vi "Fire DAQStateChanged Event_DAQ.vi"(8 "error in (no error)":errorcluster, 9 "vData":variant, 10 "DAQState":variant, 11 "DAQ":refnum<class "DAQ.lvclass">) -> (0 "error out":errorcluster, 3 "DAQ out":refnum<class "DAQ.lvclass">)   [LabVIEW 2017, in "DAQ.lvclass"]
doc: "Developed by Kevin Thompson\nkevin@thompsonengineering.net\n\nCopyright 2018-2020\nThompson Engineering, LLC"
uses:
  DAQ.lvclass
  DataTypes/TD DAQStateChanged EventData--cluster.ctl
  DataTypes/TD DAQ&TDMS State Data--cluster.ctl
  DataTypes/TD DaqState--enum.ctl
  DAQ.lvclass/DAQ.ctl
  Accessors/Get DAQ&TDMS State Data.vi
  Accessors/Set DAQ&TDMS State Data.vi
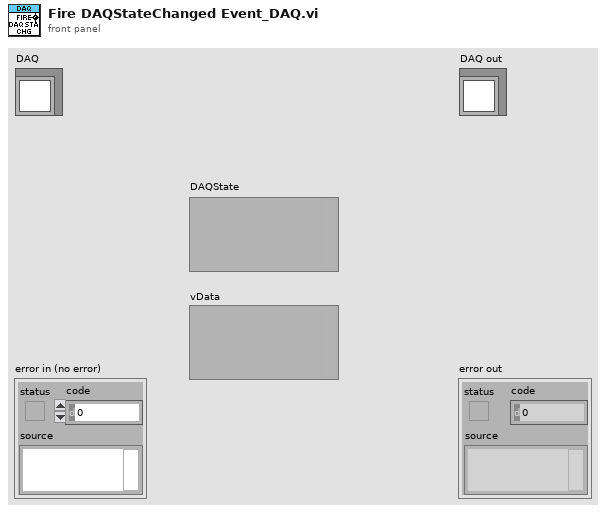
[diagram p1: front panel]
types:
  T1 = typedef "DAQ.lvclass/TD DaqState--enum.ctl" = enum16{"Unknown", "Stopped", "Running", "Error"}
  T2 = typedef "DAQ.lvclass/TD DAQStateChanged EventData--cluster.ctl" = cluster{"Time Stamp":timestamp, "OLD State Data":T3, "NEW State Data":T3}
  T3 = typedef "DAQ.lvclass/TD DAQ&TDMS State Data--cluster.ctl" = cluster{"DAQState":T1, "vData":variant}
  T4 = typedef "Type Descriptor Enumeration__ogtk.ctl" = enum8{"<Null>", "I8", "I16", "I32", "I64", "U8", "U16", "U32", "U64", "SGL", "DBL", "EXT", "CSG", "CDB", "CXT", "0x0F", "0x10", "0x11", "0x12", "0x13", "0x14", "Enum U8", "Enum U16", "Enum U32", "Enum U64", "SGL PQ", "DBL PQ", "EXT PQ", "CSG PQ", "CDB PQ", "CXT PQ", "0x1F", "0x20", "Boolean", "0x22", "0x23", "0x24", "0x25", "0x26", "0x27", "0x28", "0x29", "0x2A", "0x2B", "0x2C", "0x2D", "0x2E", "0x2F", "String", "0x31", "Path", "Pict", "0x34", "0x35", "0x36", "DAQ", "0x38", "0x39", "0x3A", "0x3B", "0x3C", "0x3D", "0x3E", "0x3F", "Array", "0x41", "0x42", "0x43", "0x44", "0x45", "0x46", "0x47", "0x48", "0x49", "0x4A", "0x4B", "0x4C", "0x4D", "0x4E", "0x4F", "Cluster", "0x51", "0x52", "Variant", "Waveform", "0x55", "0x56", "0x57", "0x58", "0x59", "0x5A", "0x5B", "0x5C", "0x5D", "0x5E", "0x5F", "0x60", "0x61", "0x62", "0x63", "0x64", "0x65", "0x66", "0x67", "0x68", "0x69", "0x6A", "0x6B", "0x6C", "0x6D", "0x6E", "0x6F", "Refnum"}
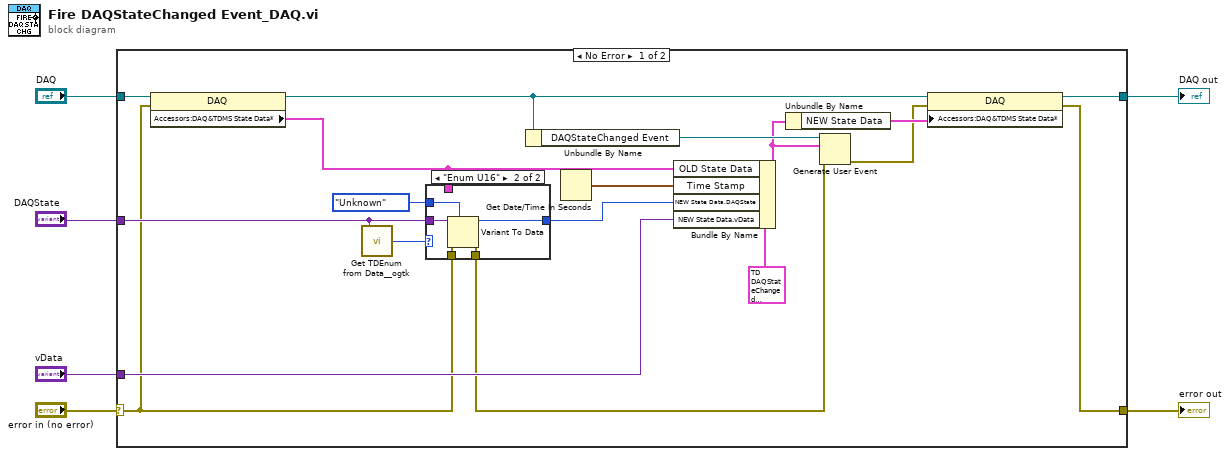
[diagram p0: block diagram]
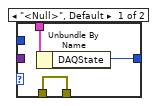
[diagram p2: hidden frame]
diagram:
  n1 = case shown="No Error" "error in (no error)" {
    selector: "error in (no error)" -> [w7 w34]
    tunnel: [w8 w34] -> w5
    tunnel: [w12 w33] -> w3
    tunnel: "DAQ" -> [w21 w33]
    tunnel: "DAQState" -> [w19 _]
    tunnel: "vData" -> [w16 _]
    frame No Error {
      n2 = property class="DAQ"(reference=w21, error in=w7) -> (reference out=w13:refnum<class "DAQ.lvclass">, "Accessors:DAQ&TDMS State Data*"=w14:T3)  [unwired: 1 out]
      n3 = call <userlib>:"Get TDEnum from Data__ogtk.vi"("Data"=w19) -> ("Type Descriptor Enumeration"=w20:T4)  [unwired: 4 in]
      n4 = case shown="\"Enum U16\"" w20 {
        tunnel: w14 -> [w27 _]
        tunnel: w19 -> [_ w32]
        tunnel: [w26 w31] -> w17
        tunnel: TD_DaqState--enum."Unknown" ("DAQState") -> [_ w30]
        tunnel: w7 -> [w25 w29]
        tunnel: [w25 w28] -> w15
        frame "<Null>", Default {
          n5 = Unbundle By Name(w27) -> ("DAQState"=w26:T1)
        }
        frame "Enum U16" {
          n6 = Variant To Data(error in=w29, type=w30, Variant=w32) -> (data=w31:T1, error out=w28:errorcluster)
        }
      }
      n7 = Unbundle By Name(w13) -> ("DAQStateChanged Event"=w24:refnum<user-event>)
      n8 = Get Date/Time In Seconds() -> (seconds since 1Jan1904=w23:timestamp)
      n9 = Bundle By Name(cluster=T2 {"Time Stamp"=timestamp(0 s since 1904-01-01), "OLD State Data"={"DAQState"=enum."Stopped", "vData"=variant}, "NEW State Data"={"DAQState"=enum."Stopped", "vData"=variant}} ("DAQStateChanged EventData"), "OLD State Data"=w14, "Time Stamp"=w23, "NEW State Data.DAQState"=w17, "NEW State Data.vData"=w16) -> (w11:T2)
      n10 = Unbundle By Name(w11) -> ("NEW State Data"=w10:T3)
      n11 = Generate User Event(user event=w24, event data cluster=w11, error in=w15) -> (error out=w9:errorcluster)  [unwired: 1 in, 1 out]
      n12 = property class="DAQ"(reference=w13, error in=w9, "Accessors:DAQ&TDMS State Data*"=w10) -> (reference out=w12:refnum<class "DAQ.lvclass">, error out=w8:errorcluster)
    }
    frame Error {
    }
  }
  "error out" <- w5
  "DAQ out" <- w3
